vi "Error Queue Count.vi"(8 "error in (no error)":errorcluster, 10 "Node In":string, 11 "VISA resource name":refnum<visa-resource-name>) -> (0 "error out":errorcluster, 1 "Error Count":i32, 2 "Node  Out":string, 3 "VISA resource name out":refnum<visa-resource-name>, 4 "Command String":string)   [LabVIEW 2009, in "Keithley 2600 Series.lvlib"]
doc: "Returns the number of entries in the instrument's error/event queue.\n\n<b>Functions and Attributes Used</b>\nerrorqueue.count"
uses:
  <instrlib>/Keithley 2600 Series/Keithley 2600 Series.lvlib
panel:
  # "(c) 2008 Keithley Instruments, Inc.  ALL RIGHTS RESERVED."
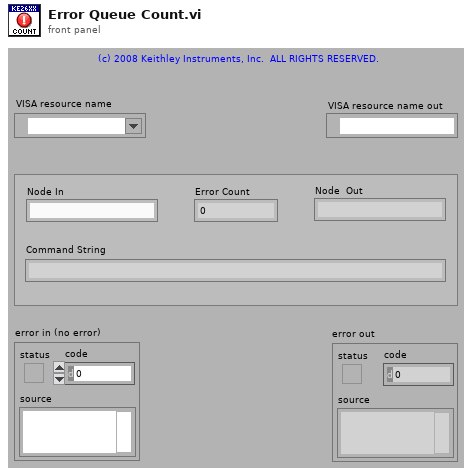
[diagram p1: front panel]
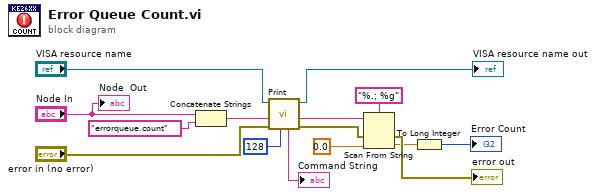
[diagram p0: block diagram]
diagram:
  n1 = Concatenate Strings("Node In", "errorqueue.count" ("command")) -> (w8:string)
  n2 = call <instrlib>:"Print.vi"("Byte Count (1024)"=u32 128, "error in (no error)"="error in (no error)", "Input"=w8, "VISA resource name"="VISA resource name") -> ("error out"=w4:errorcluster, "Output"=w5:string, "VISA resource name out"=→"VISA resource name out":refnum<visa-resource-name>, "Command String"=→"Command String":string)  [unwired: 1 in, 3 out]
  n3 = Scan From String(format string="%.; %g", input string=w5, error in=w4, default 1=0.0 ("default value 1")) -> (error out=→"error out":errorcluster, output 1=w12:dbl)  [unwired: 1 in, 2 out]
  n4 = To Long Integer(number=w12) -> (32bit integer=→"Error Count":i32)
  "Node  Out" <- "Node In"
